vi "Init.vi"(8 "error in (no error)":errorcluster, 11 "uService Template in":refnum<class "DAQ Sender.lvclass">) -> (0 "error out":errorcluster, 3 "uService Template out":refnum<class "DAQ Sender.lvclass">)   [LabVIEW 2020, in "CIRCUS_uServices.lvlib" / "DAQ Sender.lvlib" / "DAQ Sender.lvclass"]
uses:
  DAQ Sender.lvclass
  DAQ Sender.lvclass/DAQ Sender.ctl
  TALOS/TALOS_PPL.lvlibp/Ancestor/Ancestor/Ancestor.lvclass
  TALOS/TALOS_PPL.lvlibp/Father of all uServices/Father of all uServices/Father of all uServices.lvclass
  TALOS/TALOS_PPL.lvlibp
  C:/Users/marco/Documents/GitHub_Lab/CIRCUS/TALOS/TALOS_PPL.lvlibp/Father of all uServices/Father of all uServices/Father of all uServices.lvclass
  C:/Users/marco/Documents/GitHub_Lab/CIRCUS/TALOS/TALOS_PPL.lvlibp/Ancestor/Ancestor/Ancestor.lvclass
  C:/Users/marco/Documents/GitHub_Lab/CIRCUS/TALOS/Actor Framework.lvlibp/1abvi3w/vi.lib/ActorFramework/Actor/Actor.lvclass
  C:/Users/marco/Documents/GitHub_Lab/CIRCUS/CIRCUS uServices et al/DAQ Sender/DAQ Sender/DAQ Sender.lvclass
  TALOS/TALOS_PPL.lvlibp/Interfaces/DAQ Communication/DAQ Communication.lvclass
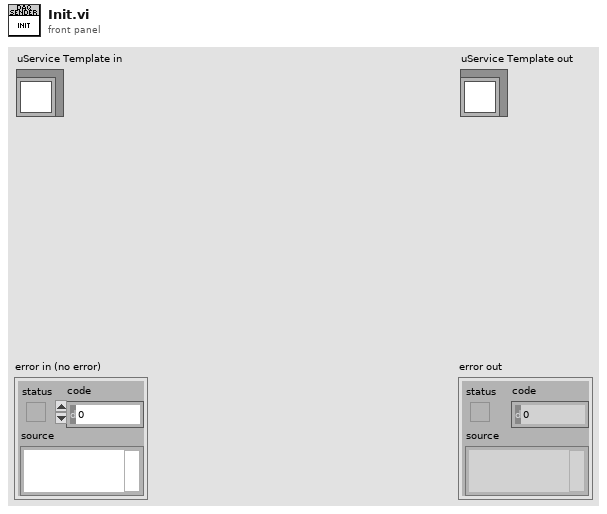
[diagram p1: front panel]
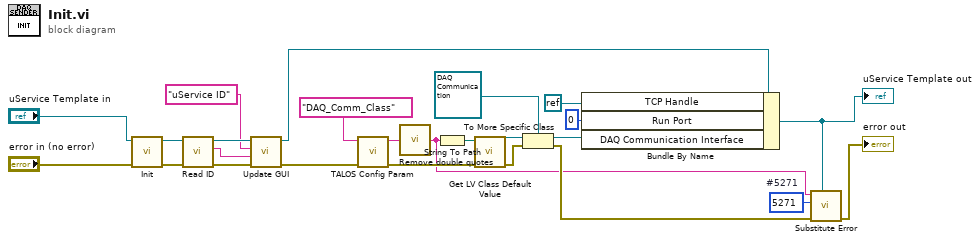
[diagram p0: block diagram]
diagram:
  w12 = 5271  # #5271
  n1 = call-parent "Init.vi"("error in (no error)"="error in (no error)", "uService Template in"="uService Template in") -> ("error out"=w21:errorcluster, "uService Template out"=w22:refnum<class "DAQ Sender.lvclass">)  [unwired: 8 in]
  n2 = call "Read ID.vi"("error in (no error)"=w21, "Ancestor in"=w22) -> ("error out"=w20:errorcluster, "ID"=w17:string, "Ancestor out"=w19:refnum<class "DAQ Sender.lvclass">)  [unwired: 7 in]
  n3 = call "Update GUI.vi"("error in (no error)"=w20, "Data"=w17, "GUI Item Name"="uService ID", "uService Template in"=w19) -> ("error out"=w1:errorcluster, "uService Template out"=w9:refnum<class "DAQ Sender.lvclass">)  [unwired: 6 in]
  n4 = call "TALOS Config Param.vi"("error in (no error)"=w1, "Parameter Name"="DAQ_Comm_Class") -> ("error out"=w25:errorcluster, "Output"=w2:string)  [unwired: 8 in]
  n5 = call "Remove double quotes.vi"("Input string"=w2) -> ("Output string"=w10:string)  [unwired: 4 in]
  n6 = String To Path(string=w10) -> (path=w16:path)
  n7 = call <vilib>:"Get LV Class Default Value.vi"("error in (no error)"=w25, "class path"=w16) -> ("error out"=w15:errorcluster, "object"=w14:refnum<class>)  [unwired: 8 in]
  n8 = To More Specific Class(target class=refnum<class "DAQ Communication.lvclass"> refnum ("DAQ Communication"), reference=w14, error in=w15) -> (specific class reference=w11:refnum<class "DAQ Communication.lvclass">, error out=w13:errorcluster)
  n9 = Bundle By Name(cluster=w9, "TCP Handle"=refnum<k0> refnum, "Run Port"=u16 0, "DAQ Communication Interface"=w11) -> (w7:refnum<class "DAQ Sender.lvclass">)
  "uService Template out" <- w7
  n10 = call "Substitute Error.vi"("LabVIEW Object"=w7, "error in (no error)"=w13, "Error Code"=w12, "Optional String"=w10) -> ("error out"=→"error out":errorcluster)  [unwired: 7 in]
